vi "WaveformCreator.vi"(6 "BusNumber":u16, 8 "error":dbl[][](array[numeric]), 9 "dt":dbl, 10 "Vestimate":cdb[][](array[numeric]), 11 "SystemVoltagesRef":cdb[][](array[numeric])) -> (1 "MagnitudeEstimate":waveform(dbl)[](array[waveform]), 2 "AngleEstimate":waveform(dbl)[](array[waveform]), 3 "TVE":waveform(dbl))   [LabVIEW 2017, in "Visualization.lvlib" / "VisualizeAppLSE.lvclass"]
uses:
  VisualizeAppLSE.lvclass
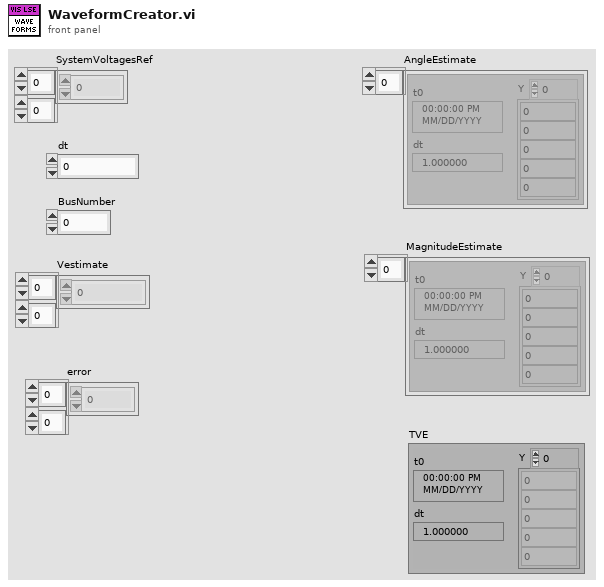
[diagram p1: front panel]
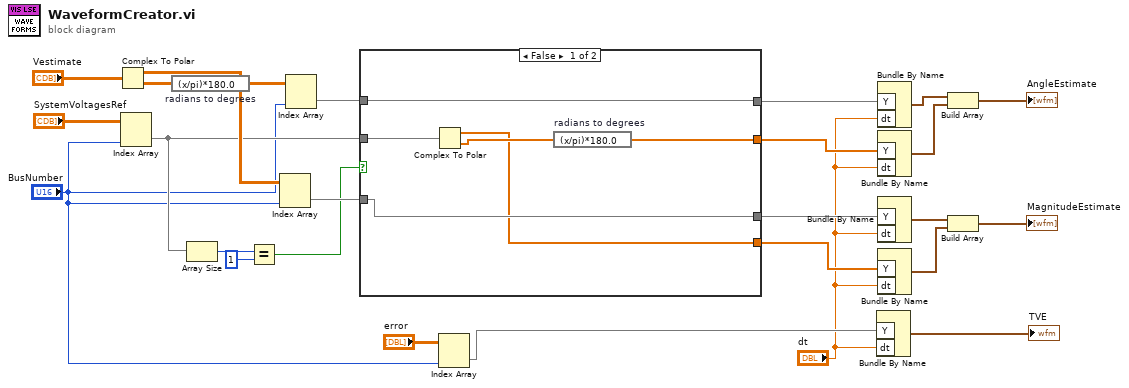
[diagram p0: block diagram]
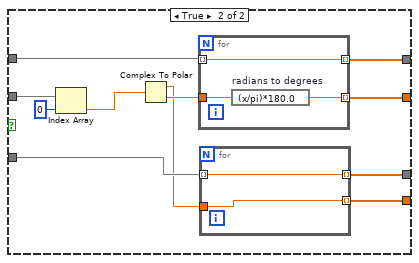
[diagram p2: hidden frame]
diagram:
  n1 = Complex To Polar(r * e^(i*theta)="Vestimate") -> (r=w17:dbl[][], theta=w26:dbl[][])
  n2 = Index Array(array="SystemVoltagesRef", index (col)="BusNumber") -> (element=w5:cdb[])  [unwired: 1 in]
  n3 = expression code="(x/pi)*180.0" "radians to degrees"(w26) -> (w16:dbl[][])
  n4 = Array Size(array=w5) -> (size(s)=w4:i32)
  n5 = Equal?(x=w4, y=1) -> (x = y?=w2:bool)
  n6 = Index Array(array=w17, index (col)="BusNumber") -> (element=w13:dbl[])  [unwired: 1 in]
  n7 = Index Array(array=w16, index (col)="BusNumber") -> (element=w6:dbl[])  [unwired: 1 in]
  n8 = case shown="False" w2 {
    tunnel: [w32 w43] -> w15
    tunnel: [w29 w42] -> w14
    tunnel: w13 -> [w31 w41]
    tunnel: [w31 w40] -> w12
    tunnel: [w28 w39] -> w11
    tunnel: w5 -> [w27 w35]
    tunnel: w6 -> [w32 w38]
    frame False {
      n9 = Complex To Polar(r * e^(i*theta)=w27) -> (r=w28:dbl[], theta=w30:dbl[])
      n10 = expression code="(x/pi)*180.0" "radians to degrees"(w30) -> (w29:dbl[])
    }
    frame True {
      n11 = Index Array(array=w35, index=0) -> (element=w34:cdb)
      n12 = Complex To Polar(r * e^(i*theta)=w34) -> (r=w36:dbl, theta=w37:dbl)
      n13 = for {
        tunnel: [w46] -> w42 mode=indexing
        tunnel: w37 -> [w47]
        tunnel: [w48] -> w43 mode=indexing
        tunnel: w38 -> [w48] mode=indexing
        n14 = expression code="(x/pi)*180.0" "radians to degrees"(w47) -> (w46:dbl)
      }
      n15 = for {
        tunnel: [w44] -> w39 mode=indexing
        tunnel: w41 -> [w45] mode=indexing
        tunnel: [w45] -> w40 mode=indexing
        tunnel: w36 -> [w44]
      }
    }
  }
  n16 = Index Array(array="error", index (col)="BusNumber") -> (element=w9:dbl[])  [unwired: 1 in]
  n17 = Bundle By Name("Y"=w9, "dt"="dt") -> (→"TVE":waveform(dbl))  [unwired: 1 in]
  n18 = Bundle By Name("Y"=w15, "dt"="dt") -> (w23:waveform(dbl))  [unwired: 1 in]
  n19 = Bundle By Name("Y"=w14, "dt"="dt") -> (w22:waveform(dbl))  [unwired: 1 in]
  n20 = Bundle By Name("Y"=w12, "dt"="dt") -> (w25:waveform(dbl))  [unwired: 1 in]
  n21 = Bundle By Name("Y"=w11, "dt"="dt") -> (w24:waveform(dbl))  [unwired: 1 in]
  n22 = Build Array(w23, w22) -> (→"AngleEstimate":waveform(dbl)[])
  n23 = Build Array(w25, w24) -> (→"MagnitudeEstimate":waveform(dbl)[])
